vi "eFGV - Stop Program.vi"(6 "State - eFGV":T1=enum."Close", 8 "error in (no error)":errorcluster, 10 "Stop Program":bool) -> (0 "error out":errorcluster, 2 "Event - Stop Program":refnum<user-event>)   [LabVIEW 2020]
uses:
  Control/State - eFGV.ctl
  <vilib>/event_ctls.llb/usereventprio.ctl
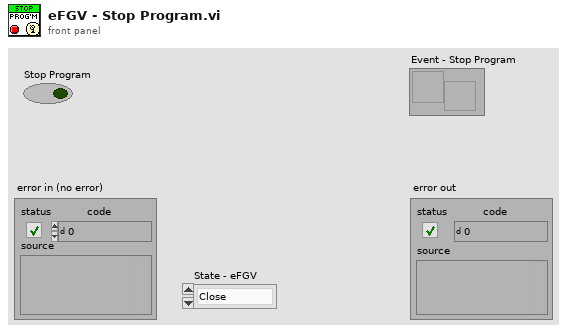
[diagram p1: front panel]
types:
  T1 = typedef "State - eFGV.ctl" = enum16{"Init", "Read", "Write", "Close"}
  T2 = typedef "usereventprio.ctl" = enum32{"high priority", "normal priority"}
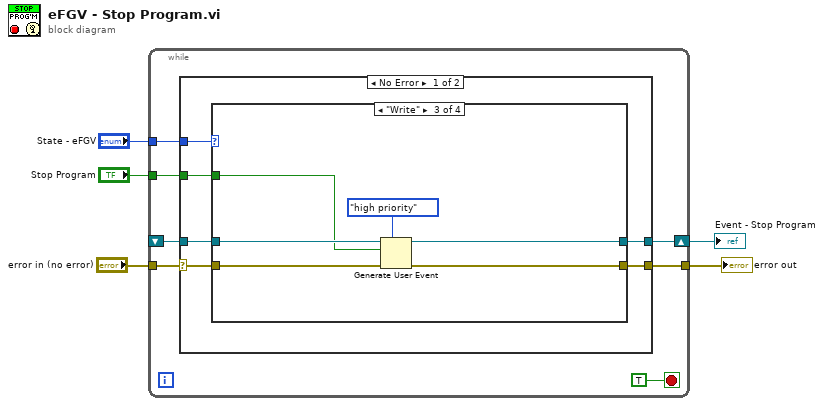
[diagram p0: block diagram]
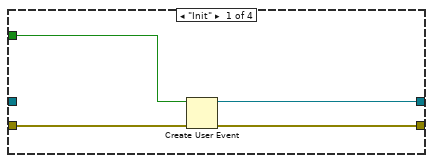
[diagram p2: hidden frame]
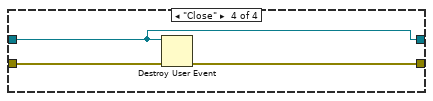
[diagram p4: hidden frame]
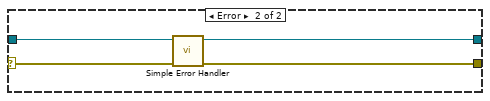
[diagram p5: hidden frame]
diagram:
  n1 = while {
    tunnel: "State - eFGV" -> [w11]
    tunnel: "error in (no error)" -> [w10]
    tunnel: [w9] -> w3
    shift-right: [w8] -> w1
    shift-left: _ -> [w7]
    tunnel: "Stop Program" -> [w6]
    stop <- TRUE stop-if-true
    n2 = case shown="No Error" w10 {
      selector: w10 -> [w17 w36]
      tunnel: w11 -> [w18 _]
      tunnel: [w16 w34] -> w9
      tunnel: [w15 w35] -> w8
      tunnel: w7 -> [w14 w35]
      tunnel: w6 -> [w13 _]
      frame No Error {
        n3 = case shown="\"Write\"" w18 {
          tunnel: w17 -> [w22 w24 w30 w33]
          tunnel: [w21 w24 w29 w32] -> w16
          tunnel: [w20 w23 w28 w31] -> w15
          tunnel: w14 -> [_ w23 w27 w31]
          tunnel: w13 -> [w19 _ w26 _]
          frame "Init" {
            n4 = Create User Event(user event datatype=w19, error in=w22) -> (user event=w20:refnum<user-event>, error out=w21:errorcluster)
          }
          frame "Read", Default {
          }
          frame "Write" {
            n5 = Generate User Event(priority (normal)=usereventprio."high priority", user event=w27, event data cluster=w26, error in=w30) -> (user event out=w28:refnum<user-event>, error out=w29:errorcluster)
          }
          frame "Close" {
            n6 = Destroy User Event(user event=w31, error in=w33) -> (error out=w32:errorcluster)
          }
        }
      }
      frame Error {
        n7 = call <vilib>:"Simple Error Handler.vi"("error in (no error)"=w36) -> ("error out"=w34:errorcluster)  [unwired: 4 in, 4 out]
      }
    }
  }
  "error out" <- w3
  "Event - Stop Program" <- w1
